vi "field setpoint(SubVI).vi"(0 "Filed 2":dbl=300.0, 1 "Field":dbl=300.0, 3 "Rate":dbl=10.0, 4 "Mode":i32(ring) items=["Persistent", "Driven"], 5 "Instrument Ref":refnum<k24>, 6 "data":refnum<queue>, 7 "Delay":dbl, 9 "steps number":i32, 11 "Approach":i32(ring) items=["FastSettle", "NoOvershoot"], 12 "ch str":string, 13 "Resource In":refnum<visa-resource-name>, 15 "config":refnum<queue>) -> (8 "错误输出":errorcluster)   [LabVIEW 2019, in "old.lvlib"]
uses:
  old.lvlib
  SubVI.lvlib
  config.ctl
  lib/QDInstrument.dll
  <vilib>/NI/Modbus Library/API/Master/Modbus Master.lvclass
  Instrument.ctl
panel:
  out "数组":dbl[](array[numeric])
  # "(真是通道1，假是通道2)"
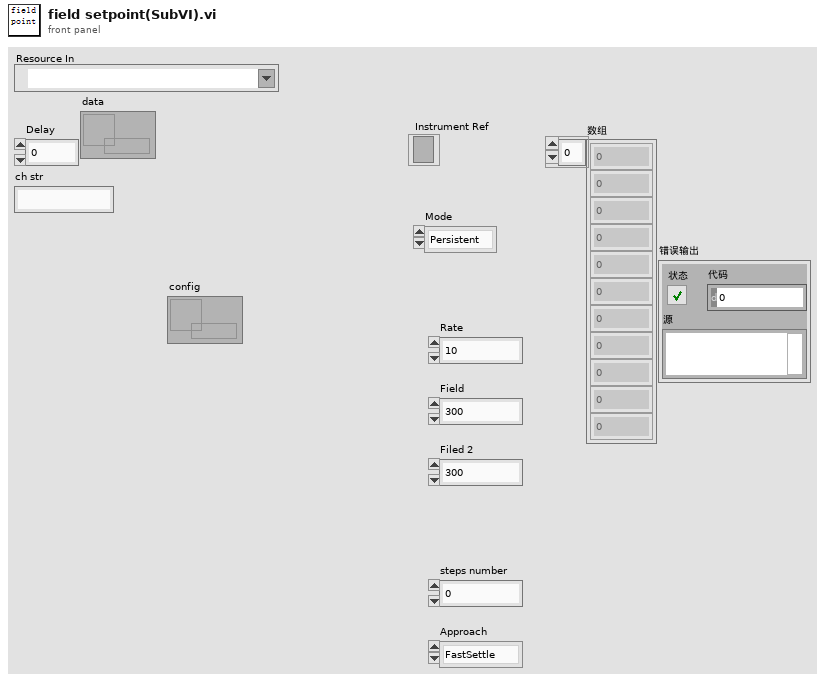
[diagram p1: front panel]
types:
  T1 = typedef "config.ctl" = cluster{"initialize":string, "6221":cluster{"6221 Resource":refnum<visa-resource-name>, "Delta status":bool}, "7001":cluster{"Ch":bool}, "SR830+6221":cluster{"source":u16, "阻抗":dbl, "量程入 4":i32, "量程入 3":i32, "量程入 2":i32, "量程入 1":i32, "电流":dbl, "SR830 2":bool, "SR830 3":bool, "SR830 4":bool, "SR830 1":bool, "VISA 1":refnum<visa-resource-name>, "VISA 2":refnum<visa-resource-name>, "VISA 3":refnum<visa-resource-name>, "VISA 4":refnum<visa-resource-name>, "量程":enum16{"量程每次测量会判定", "量程不变为设定值"}}, "2400":cluster{"2400":bool, "VISA":refnum<visa-resource-name>}, "ch":cluster{"ch str":string, "ch1":bool, "ch2":bool, "布尔":bool}, "error":bool, "数据文件路径":path, "log":cluster{"log路径":path, "log interval":dbl}, "Instrument":T2}
  T2 = typedef "Instrument.ctl" = cluster{"335 Resource":refnum<visa-resource-name>, "Input (0:A)":u16, "Instrument Type":i32, "quantum design":refnum<k24>, "Heater Output (1:1)":u16, "335state":refnum<vi>, "semaphore":T3, "TCP master instance":refnum<class "Modbus Master.lvclass">}
  T3 = typedef "Semaphore RefNum" = refnum<k1>
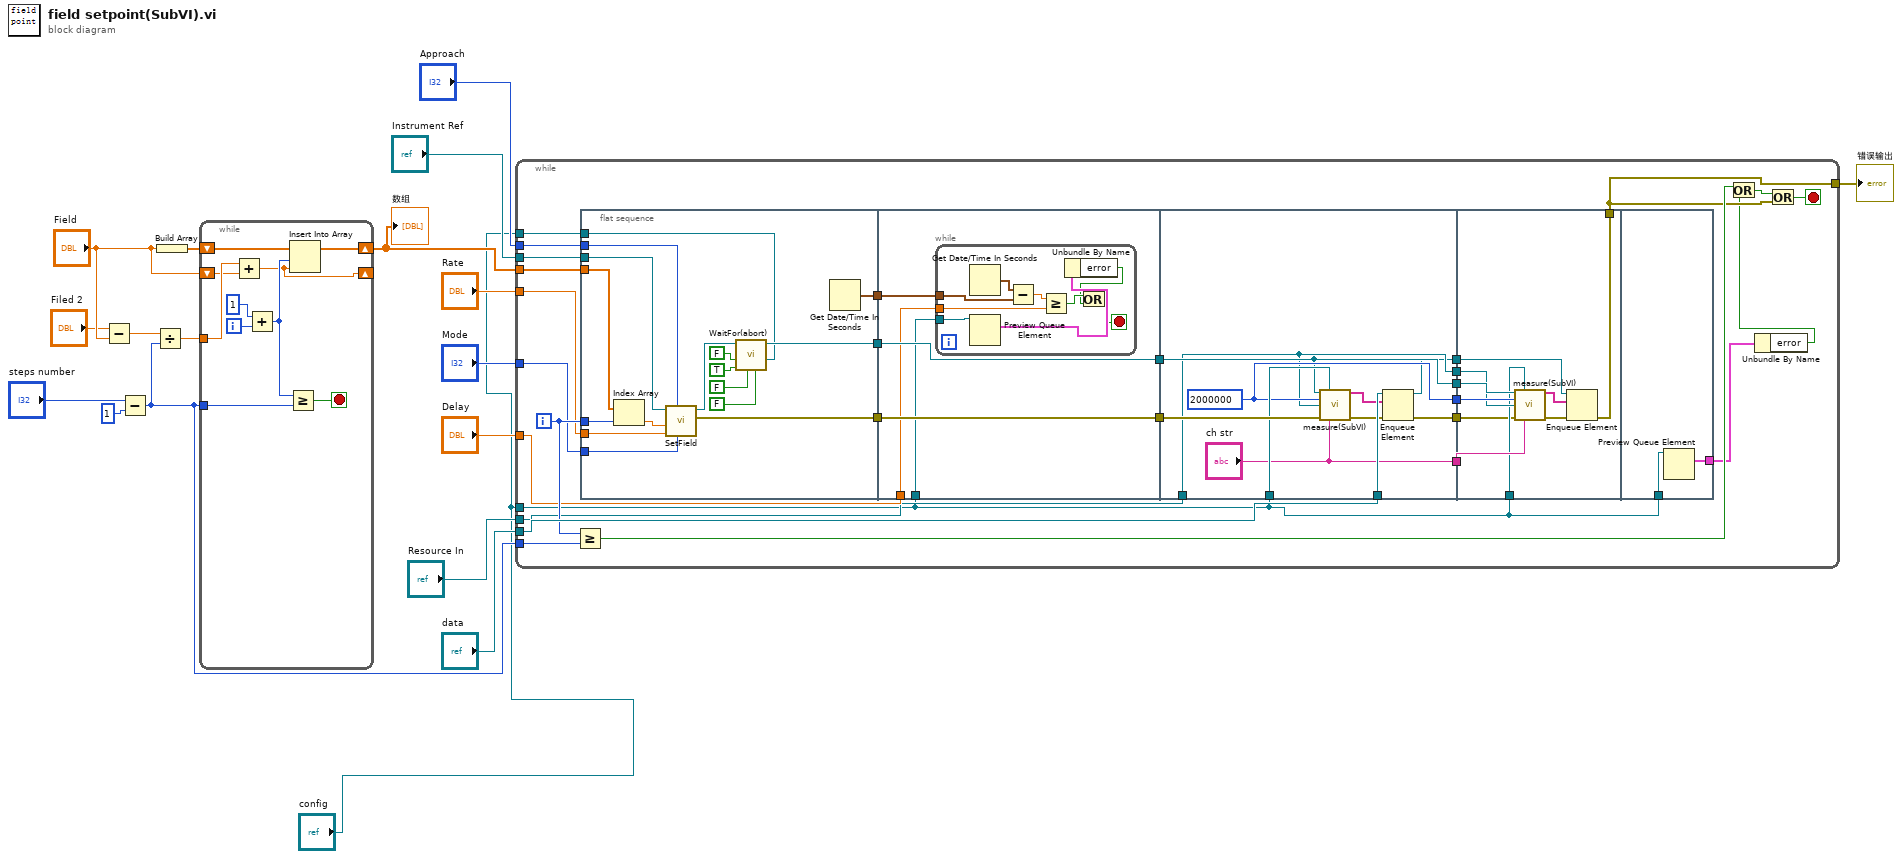
[diagram p0: block diagram]
diagram:
  n1 = Subtract(x="Filed 2", y="Field") -> (x-y=w15:dbl)
  n2 = Subtract(x="steps number", y=1) -> (x-y=w5:i32)
  n3 = Divide(x=w15, y=w5) -> (x/y=w17:dbl)
  n4 = Build Array("Field") -> (w16:dbl[])
  n5 = while {
    shift-right: [w28] -> w10
    shift-left: w16 -> [w27]
    tunnel: w17 -> [w22]
    tunnel: w5 -> [w21]
    shift-right: [w20] -> _
    shift-left: "Field" -> [w19]
    i -> [w26]
    stop <- w23 stop-if-true
    n6 = Add(x=w22, y=w19) -> (x+y=w20:dbl)
    n7 = Add(x=1, y=w26) -> (x+y=w24:i32)
    n8 = Greater Or Equal?(x=w24, y=w21) -> (x >= y?=w23:bool)
    n9 = Insert Into Array(array=w27, index=w24, new element=w20) -> (w28:dbl[])
  }
  "数组" <- w10
  n10 = while {
    tunnel: w5 -> [w55]
    tunnel: "data" -> [w57]
    tunnel: "config" -> [w34]
    tunnel: "Mode" -> [w53]
    tunnel: "Approach" -> [w52]
    tunnel: "Rate" -> [w51]
    tunnel: "Instrument Ref" -> [w50]
    tunnel: w10 -> [w49]
    tunnel: "config" -> [w48]
    tunnel: [w31] -> w8
    tunnel: "Delay" -> [w40]
    tunnel: "Resource In" -> [w39]
    i -> [w54]
    stop <- w46 stop-if-true
    n11 = Greater Or Equal?(x=w54, y=w55) -> (x >= y?=w56:bool)
    n12 = flat-sequence {
      tunnel: [w65] -> w45
      tunnel: w54 -> [w68]
      tunnel: w53 -> [w72]
      tunnel: w52 -> [w71]
      tunnel: w51 -> [w70]
      tunnel: w50 -> [w67]
      tunnel: w49 -> [w69]
      tunnel: w48 -> [w60]
      tunnel: [w59] -> w43
      tunnel: [w58] -> w41
      tunnel: w45 -> [w78]
      tunnel: [w78] -> w44
      tunnel: w43 -> [w77]
      tunnel: [w77] -> w42
      tunnel: w41 -> [w76]
      tunnel: w40 -> [w75]
      tunnel: w34 -> [w74]
      tunnel: w44 -> [w92]
      tunnel: w57 -> [w98]
      tunnel: w34 -> [w95]
      tunnel: w42 -> [w96]
      tunnel: w39 -> [w91]
      tunnel: [w93] -> w38
      tunnel: [w92] -> w37
      tunnel: [w91] -> w36
      tunnel: ["ch str"] -> w35
      tunnel: [w89] -> w33
      tunnel: [w88] -> w32
      tunnel: w38 -> [w108]
      tunnel: w37 -> [w107]
      tunnel: w36 -> [w106]
      tunnel: w35 -> [w105]
      tunnel: w34 -> [w104]
      tunnel: w33 -> [w103]
      tunnel: w32 -> [w100]
      tunnel: [w99] -> w31
      tunnel: w34 -> [w110]
      tunnel: [w109] -> w30
      frame #0 {
        n13 = Index Array(array=w69, index=w68) -> (element=w73:dbl)
        n14 = call "SetField.vi"("Mode"=w72, "Approach"=w71, "Rate"=w70, "Field"=w73, "Instrument Ref In"=w67) -> ("error out"=w59:errorcluster, "Instrument Ref Out"=w66:refnum<k24>)  [unwired: 2 in, 1 out]
        n15 = call "WaitFor(abort).vi"("config"=w60, "Wait For Chamber"=FALSE, "Wait For Position"=FALSE, "Wait For Field"=TRUE, "Wait For Temperature"=FALSE, "Instrument Ref In"=w66) -> ("Instrument Ref Out"=w65:refnum<k24>)  [unwired: 4 in, 1 out]
        n16 = Get Date/Time In Seconds() -> (seconds since 1Jan1904=w58:timestamp)
      }
      frame #1 {
        n17 = while {
          tunnel: w76 -> [w86]
          tunnel: w75 -> [w84]
          tunnel: w74 -> [w82]
          stop <- w80 stop-if-true
          n18 = Get Date/Time In Seconds() -> (seconds since 1Jan1904=w87:timestamp)
          n19 = Preview Queue Element(queue=w82) -> (element=w81:T1)  [unwired: 2 in, 3 out]
          n20 = Subtract(x=w87, y=w86) -> (x-y=w85:dbl)
          n21 = Greater Or Equal?(x=w85, y=w84) -> (x >= y?=w83:bool)
          n22 = Unbundle By Name(w81) -> ("error"=w79:bool)
          n23 = Or(x=w83, y=w79) -> (x .or. y?=w80:bool)
        }
      }
      frame #2 {
        w93 = u32 2000000 ("Timeout (20000 ms)")
        n24 = call "measure(SubVI).vi"(0:w92, "config"=w95, 5:w93, 7:w91, "error in (no error)"=w96, 12:"ch str") -> ("data"=w97:string[], "error out"=w94:errorcluster)  [unwired: 8 in]
        n25 = Enqueue Element(queue=w98, element=w97, error in (no error)=w94) -> (queue out=w89:refnum<queue>, error out=w88:errorcluster)  [unwired: 1 in, 1 out]
      }
      frame #3 {
        n26 = call "measure(SubVI).vi"(0:w107, "config"=w104, 5:w108, 7:w106, "error in (no error)"=w100, 12:w105) -> ("data"=w102:string[], "error out"=w101:errorcluster)  [unwired: 8 in]
        n27 = Enqueue Element(queue=w103, element=w102, error in (no error)=w101) -> (error out=w99:errorcluster)  [unwired: 1 in, 2 out]
      }
      frame #4 {
        n28 = Preview Queue Element(queue=w110) -> (element=w109:T1)  [unwired: 2 in, 3 out]
      }
    }
    n29 = Unbundle By Name(w30) -> ("error"=w29:bool)
    n30 = Or(x=w56, y=w29) -> (x .or. y?=w47:bool)
    n31 = Or(x=w47, y=w31) -> (x .or. y?=w46:bool)
  }
  "错误输出" <- w8
